vi "GetExecutableConfigurationFilePath.vi"(8 "Error In":errorcluster, 10 "Application Name":string, 11 "VI Path":path) -> (0 "Error Out":errorcluster, 3 "Executable Config File Path":path)   [LabVIEW 2012, in "LV-Utilities.lvlib"]
uses:
  LV-Utilities.lvlib
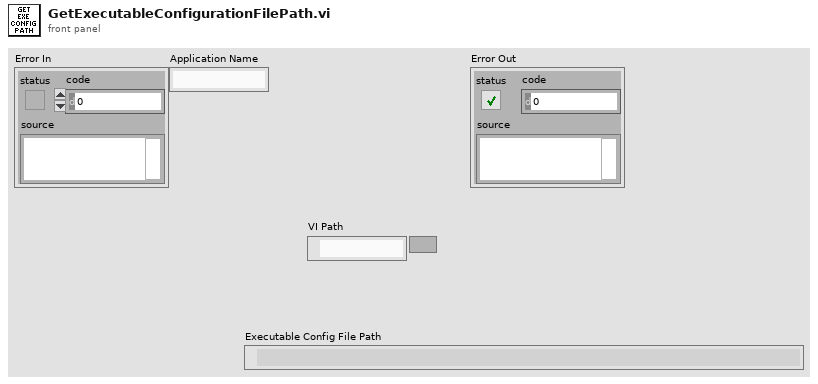
[diagram p1: front panel]
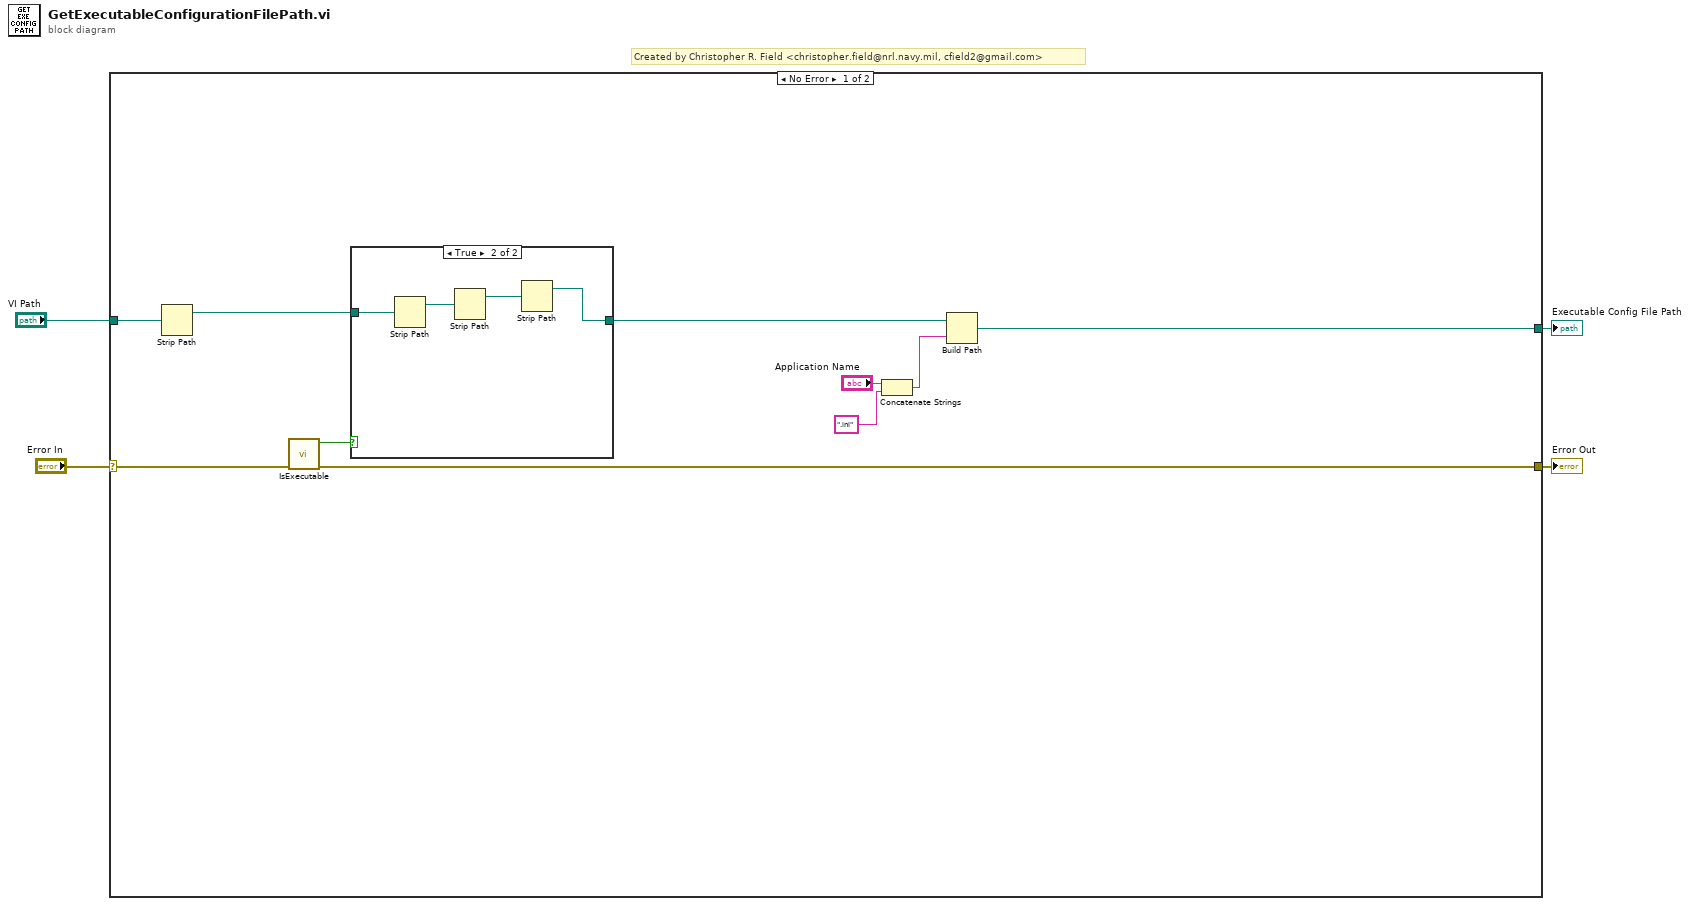
[diagram p0: block diagram]
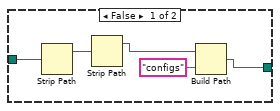
[diagram p2: hidden frame]
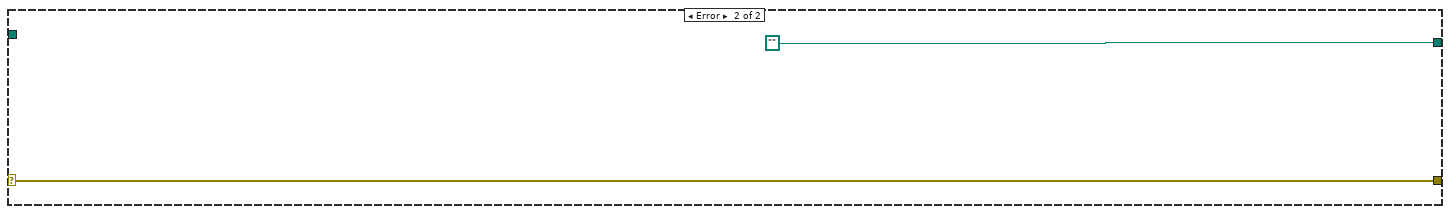
[diagram p3: hidden frame]
diagram:
  # "Created by Christopher R. Field <christopher.field@nrl.navy.mil, cfield2@gmail.com>"
  n1 = case shown="No Error" "Error In" {
    selector: "Error In" -> [w10 w24]
    tunnel: "VI Path" -> [w14 _]
    tunnel: [w8 w24] -> w2
    tunnel: [w7 path ""] -> w1
    frame No Error {
      n2 = Strip Path(path=w14) -> (stripped path=w13:path)  [unwired: 1 out]
      n3 = call "IsExecutable.vi"("Error In"=w10) -> ("Error Out"=w8:errorcluster, "Executable?"=w12:bool)  [unwired: 9 in]
      n4 = case shown="True" w12 {
        tunnel: w13 -> [w18 w23]
        tunnel: [w17 w20] -> w11
        frame False {
          n5 = Strip Path(path=w18) -> (stripped path=w16:path)  [unwired: 1 out]
          n6 = Strip Path(path=w16) -> (stripped path=w15:path)  [unwired: 1 out]
          n7 = Build Path(base path=w15, name or relative path="configs") -> (appended path=w17:path)
        }
        frame True {
          n8 = Strip Path(path=w23) -> (stripped path=w22:path)  [unwired: 1 out]
          n9 = Strip Path(path=w22) -> (stripped path=w21:path)  [unwired: 1 out]
          n10 = Strip Path(path=w21) -> (stripped path=w20:path)  [unwired: 1 out]
        }
      }
      n11 = Concatenate Strings("Application Name", ".ini" ("name or relative path")) -> (w6:string)
      n12 = Build Path(base path=w11, name or relative path=w6) -> (appended path=w7:path)
    }
    frame Error {
    }
  }
  "Error Out" <- w2
  "Executable Config File Path" <- w1
